vi "gyroLoop.vi"() -> (2 "Facing":dynamicdata(graph), 3 "Velocities":cluster{dbl, dbl, dbl}(graph))   [LabVIEW 2016]
uses:
  GLOBALS.vi
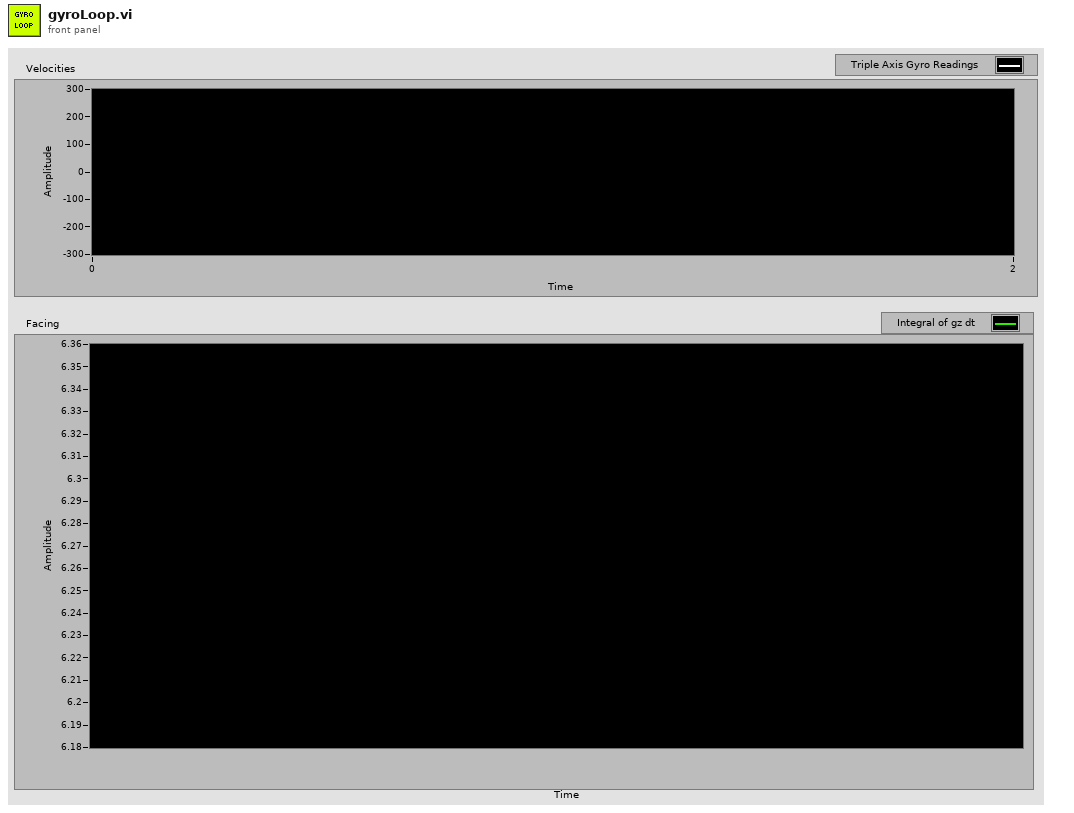
[diagram p1: front panel]
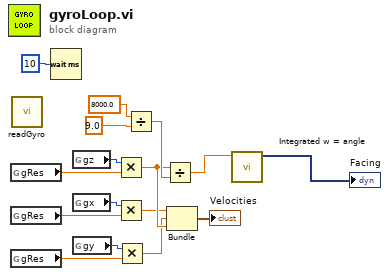
[diagram p0: block diagram]
diagram:
  n1 = global read "GLOBALS.vi" "gRes"() -> (w4:dbl)
  n2 = global read "GLOBALS.vi" "gRes"() -> (w5:dbl)
  n3 = global read "GLOBALS.vi" "gRes"() -> (w6:dbl)
  n4 = call "readGyro.vi"() -> ()  [unwired: 12 in]
  n5 = Wait (ms)(milliseconds to wait=u32 10) -> ()  [unwired: 1 out]
  n6 = global read "GLOBALS.vi" "gz"() -> (w12:i16)
  n7 = global read "GLOBALS.vi" "gx"() -> (w9:i16)
  n8 = global read "GLOBALS.vi" "gy"() -> (w7:i16)
  n9 = Multiply(x=w12, y=w4) -> (x*y=w11:dbl)
  n10 = Multiply(x=w9, y=w5) -> (x*y=w10:dbl)
  n11 = Multiply(x=w7, y=w6) -> (x*y=w8:dbl)
  n12 = Divide(x=8000.0, y=9.0) -> (x/y=w14:dbl)
  n13 = Divide(x=w11, y=w14) -> (x/y=w13:dbl)
  n14 = Bundle(w10, w8, w11) -> (→"Velocities":cluster{dbl, dbl, dbl})  [unwired: 1 in]
  n15 = call "Integrated w = angle"("Signals"=w13) -> ("Result"=→"Facing":dynamicdata)  [unwired: 5 in, 1 out]
